vi "getLUT.vi"() -> ()   [LabVIEW 2012]
panel:
  in  "Number of Entries in LUT":i32=2048
  out "Init Data Out":u32[](array[numeric])
  in  "Frequency":dbl=1000.0
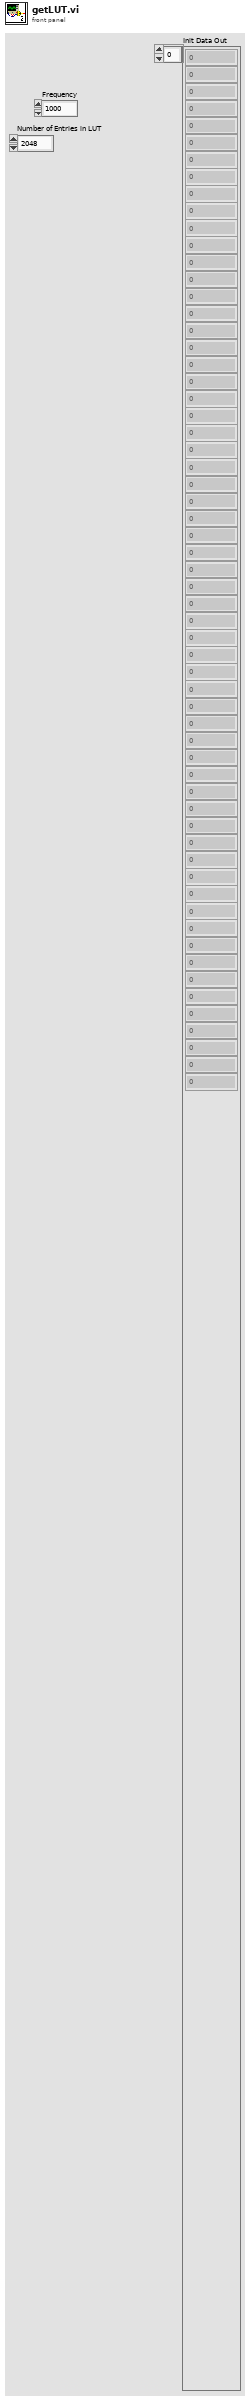
[diagram p1: front panel]
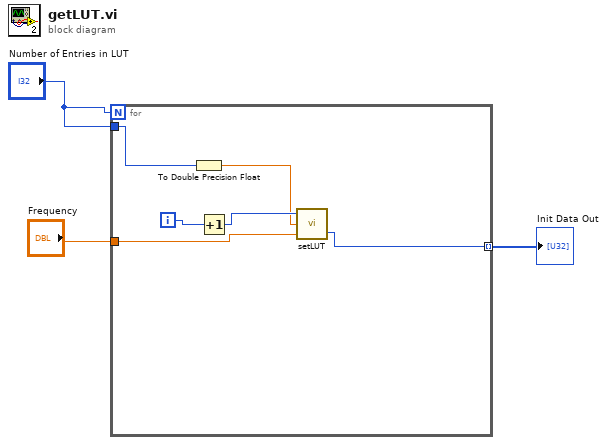
[diagram p0: block diagram]
diagram:
  n1 = for {
    N: "Number of Entries in LUT" -> [_]
    tunnel: "Frequency" -> [w4]
    tunnel: "Number of Entries in LUT" -> [w7]
    tunnel: [w8] -> w2 mode=indexing
    i -> [w9]
    n2 = To Double Precision Float(number=w7) -> (double precision float=w5:dbl)
    n3 = Increment(x=w9) -> (x+1=w6:i32)
    n4 = call "setLUT.vi"("Frequency"=w4, "Number of entries in LUT"=w5, "Count"=w6) -> ("Ticks to wait"=w8:u32)  [unwired: 1 out]
  }
  "Init Data Out" <- w2
